vi "Init Ring Acquisition.vi"(8 "error in (no error)":errorcluster, 10 "Ring Buffer Size":u32, 11 "ICamera IR in":refnum<class "ICamera.lvclass">) -> (0 "error out":errorcluster, 3 "I Camera IR out":refnum<class "ICamera.lvclass">)   [LabVIEW 2023, in "ICamera.lvclass"]
uses:
  ICamera.lvclass
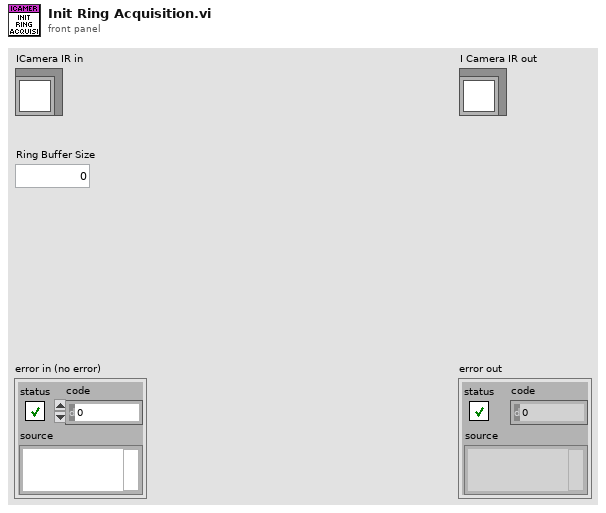
[diagram p1: front panel]
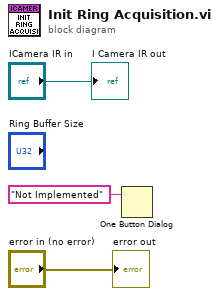
[diagram p0: block diagram]
diagram:
  n1 = One Button Dialog(message="Not Implemented") -> ()  [unwired: 1 in, 1 out]
  "error out" <- "error in (no error)"
  "I Camera IR out" <- "ICamera IR in"
